vi "Remove Header.vi"(8 "error in (no error)":errorcluster, 10 "header":string, 11 "httpHeaders in":refnum<class "httpHeaders.lvclass">) -> (0 "error out":errorcluster, 3 "httpHeaders out":refnum<class "httpHeaders.lvclass">)   [LabVIEW 2020, in "httpClient.lvlib" / "httpHeaders.lvclass"]
uses:
  httpHeaders.lvclass
  httpHeaders.lvclass/httpHeaders.ctl
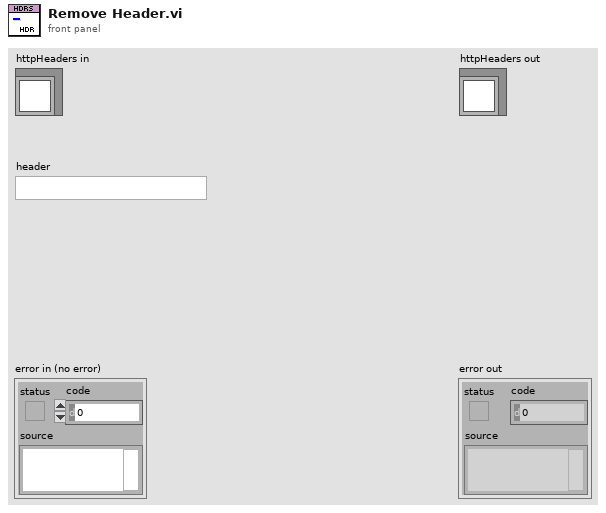
[diagram p1: front panel]
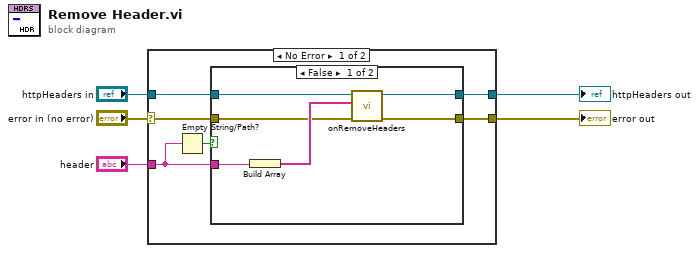
[diagram p0: block diagram]
diagram:
  n1 = case shown="No Error" "error in (no error)" {
    selector: "error in (no error)" -> [w11 w21]
    tunnel: [w10 w21] -> w4
    tunnel: [w9 w20] -> w2
    tunnel: "httpHeaders in" -> [w8 w20]
    tunnel: "header" -> [w7 _]
    frame No Error {
      n2 = Empty String/Path?(string/path=w7) -> (empty?=w6:bool)
      n3 = case shown="False" w6 {
        tunnel: w11 -> [w12 w18]
        tunnel: [w13 w18] -> w10
        tunnel: [w14 w19] -> w9
        tunnel: w8 -> [w17 w19]
        tunnel: w7 -> [w16 _]
        frame False {
          n4 = Build Array(w16) -> (w15:string[])
          n5 = call-dynamic "onRemoveHeaders.vi"("error in (no error)"=w12, "headers (empty: all)"=w15, "httpHeaders in"=w17) -> ("error out"=w13:errorcluster, "httpHeaders out"=w14:refnum<class "httpHeaders.lvclass">)  [unwired: 7 in]
        }
        frame True {
        }
      }
    }
    frame Error {
    }
  }
  "error out" <- w4
  "httpHeaders out" <- w2
